vi "1.2.1.1-VectorNav Read Write.vi"() -> ()   [LabVIEW 2010]
uses:
  <vilib>/rvi/DataTransferAndStorage/Container/XNode/niFpgaContainer.xnode
  <vilib>/rvi/DataTransferAndStorage/Container/Common/niFpgaContainerMethod.ctl
  <vilib>/rvi/DataTransferAndStorage/Container/Common/niFpgaTransferTypeControl.ctl
  <vilib>/eio/EIOMethodNode/EIOMethodNode.xnode
  <vilib>/rvi/eio/nirviEIOMethodImplementation/nirviEIOMethodImplementation.xnode
  <vilib>/rvi/eio/common/nirviEmuClasses.ctl
  1.0-Hindbrain Global.vi
  <vilib>/rvi/interface/RandomDataEmulation/nirviRandomDataFPGAFIFO.vi
  <vilib>/rvi/interface/RandomDataEmulation/niFpgaRandomDataHandleErrors.vi
  <vilib>/rvi/eio/common/nirviEmuTemplateMethod_noerrors.vi
panel:
  out "Status":enum16{"Waiting", "Reading", "Done"}(ring)
  in  "Stop Read":bool
  in  "Stop Write":bool
  out "Data":u8
  out "Element":u8
  out "Write Timeout?":bool
  out "Read from FIFOTimeout?":bool
  out "Read Timeout?":bool
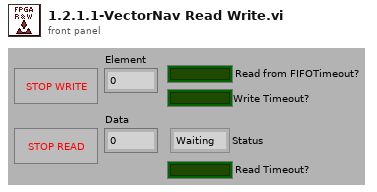
[diagram p1: front panel]
types:
  T1 = typedef "niFpgaContainerMethod.ctl" = enum16{"<none>", "write", "read", "clear", "getNumberOfElementsToWrite", "getNumberOfElementsToRead", "enable", "disable", "flushAndDisable", "getStreamState", "readA", "readB", "dramWrite", "dramWriteWithByteEnables", "dramRequestData", "dramRetrieveData"}
  T2 = typedef "niFpgaTransferTypeControl.ctl" = enum16{"Target-Scoped", "Host to Target - DMA", "Target to Host - DMA", "Peer to Peer Reader", "Peer to Peer Writer", "Bidirectional"}
  T3 = typedef "nirviEmuClasses.ctl" = enum16{"IO Read", "IO Write", "Method", "Property Read", "Property Write"}
  T4 = typedef "2.7-Sense Queries Typedef.ctl" = cluster{"VectorNav Query":bool}
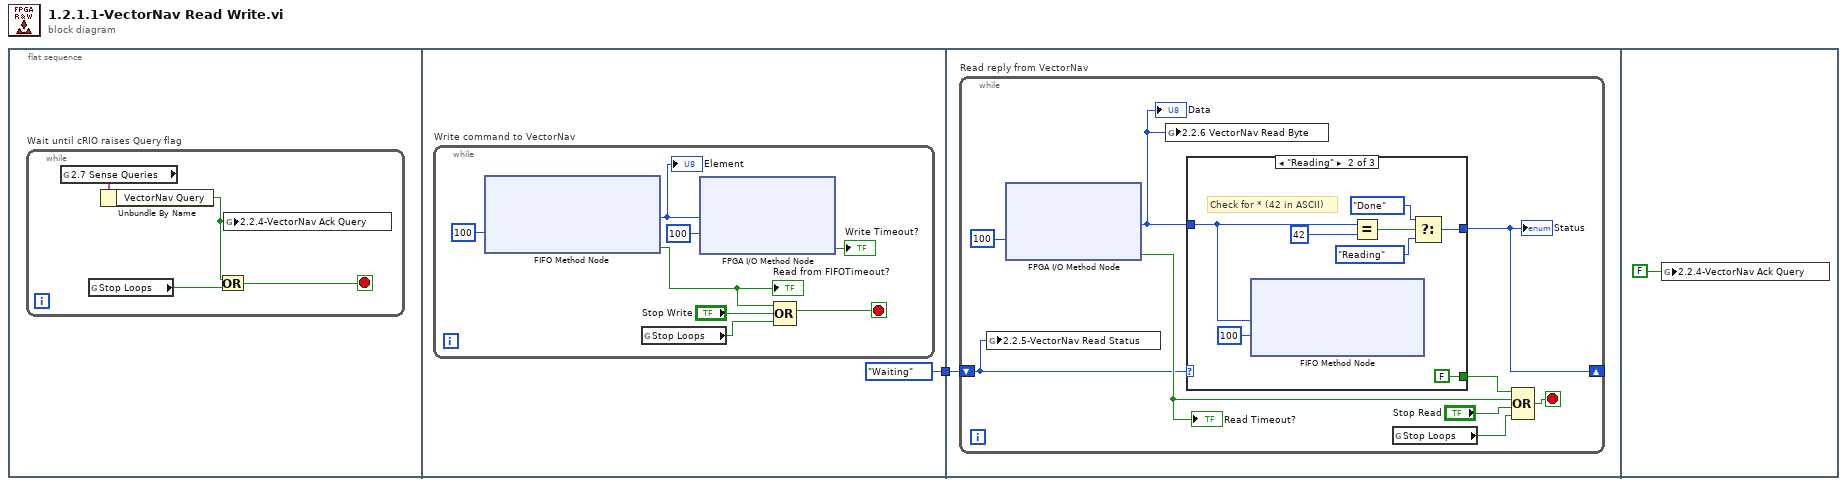
[diagram p0: block diagram]
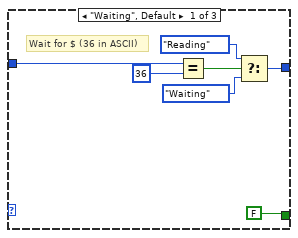
[diagram p2: hidden frame]
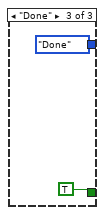
[diagram p3: hidden frame]
diagram:
  n1 = flat-sequence {
    tunnel: [enum16{"Waiting", "Reading", "Done"}."Waiting"] -> w1
    tunnel: w1 -> [w69]
    frame #0 {
      n2 = while "Wait until cRIO raises Query flag" {
        stop <- w4 stop-if-true
        n3 = global read "1.0-Hindbrain Global.vi" "2.7 Sense Queries"() -> (w5:T4)
        n4 = global read "1.0-Hindbrain Global.vi" "Stop Loops"() -> (w3:bool)
        n5 = Unbundle By Name(w5) -> ("VectorNav Query"=w2:bool)
        n6 = Or(x=w2, y=w3) -> (x .or. y?=w4:bool)
        n7 = global write "1.0-Hindbrain Global.vi" "2.2.4-VectorNav Ack Query"(w2) -> ()
      }
    }
    frame #1 {
      n8 = while "Write command to VectorNav" {
        stop <- w9 stop-if-true
        n9 = xnode ("FIFO Method Node")("Timeout"=100) -> ("Element"=w14:u8, "Timed Out?"=w10:bool)  [unwired: 1 in, 1 out]
        "Read from FIFOTimeout?" <- w10
        "Element" <- w14
        n10 = global read "1.0-Hindbrain Global.vi" "Stop Loops"() -> (w7:bool)
        n11 = xnode "FPGA I/O Method Node"("Data"=w14, "Timeout (ms)"=100) -> ("Timed Out"=→"Write Timeout?":bool)  [unwired: 1 in, 1 out]
        n12 = Compound Arithmetic op=OR(w10, "Stop Write", w7) -> (w9:bool)
      }
    }
    frame #2 {
      n13 = while "Read reply from VectorNav" {
        shift-right: [w76] -> _
        shift-left: w69 -> [w71]
        stop <- w77 stop-if-true
        n14 = global write "1.0-Hindbrain Global.vi" "2.2.5-VectorNav Read Status"(w71) -> ()
        n15 = xnode "FPGA I/O Method Node"("Timeout (ms)"=100) -> ("Data"=w70:u8, "Timed Out"=w74:bool)  [unwired: 1 in, 1 out]
        "Read Timeout?" <- w74
        "Data" <- w70
        n16 = global write "1.0-Hindbrain Global.vi" "2.2.6 VectorNav Read Byte"(w70) -> ()
        n17 = case shown="\"Reading\"" w71 {
          tunnel: w70 -> [w85 w87 _]
          tunnel: [w80 w88 enum16{"Waiting", "Reading", "Done"}."Done"] -> w76
          tunnel: [FALSE ("Stop") FALSE ("Stop") TRUE ("Stop")] -> w75
          frame "Waiting", Default {
            # "Wait for $ (36 in ASCII)"
            n18 = Equal?(x=w85, y=u8 36) -> (x = y?=w83:bool)
            n19 = Select(t=enum16{"Waiting", "Reading", "Done"}."Reading", s=w83, f=enum16{"Waiting", "Reading", "Done"}."Waiting") -> (s? t:f=w80:enum16{"Waiting", "Reading", "Done"})
          }
          frame "Reading" {
            # "Check for * (42 in ASCII)"
            n20 = xnode ("FIFO Method Node")("Element"=w87, "Timeout"=100) -> ()  [unwired: 1 in, 2 out]
            n21 = Equal?(x=w87, y=u8 42) -> (x = y?=w91:bool)
            n22 = Select(t=enum16{"Waiting", "Reading", "Done"}."Done", s=w91, f=enum16{"Waiting", "Reading", "Done"}."Reading") -> (s? t:f=w88:enum16{"Waiting", "Reading", "Done"})
          }
          frame "Done" {
          }
        }
        "Status" <- w76
        n23 = global read "1.0-Hindbrain Global.vi" "Stop Loops"() -> (w72:bool)
        n24 = Compound Arithmetic op=OR(w75, w74, "Stop Read", w72) -> (w77:bool)
      }
    }
    frame #3 {
      n25 = global write "1.0-Hindbrain Global.vi" "2.2.4-VectorNav Ack Query"(FALSE ("2.2.4-VectorNav Query")) -> ()
    }
  }
